vi "data_process_packet.vi"(6 "Sensor Lookup Indices":i32[](array[numeric]), 7 "Gains":dbl[](array[numeric])=[1.502, 1.502, 2.42], 8 "error in (no error)":errorcluster, 10 "No. Sensors":i32=128, 11 "Binary Input Data":string) -> (0 "error out":errorcluster, 1 "Raw Sensors N x XYZ":dbl[][](array[numeric]), 2 "Raw Sensors (Flattened)":i16[](array[numeric]), 3 "Time":u32, 4 "Sensors (uT)":dbl[][](array[numeric]))   [LabVIEW 2018]
panel:
  in  "LE?":bool=TRUE
  out "index of element":i32
  in  "threshold":dbl
  out "Z data":dbl[](graph)
  in  "byte order (0:big-endian, network order)":T1(ring)=enum."little-endian"
  out "Time Packet":string
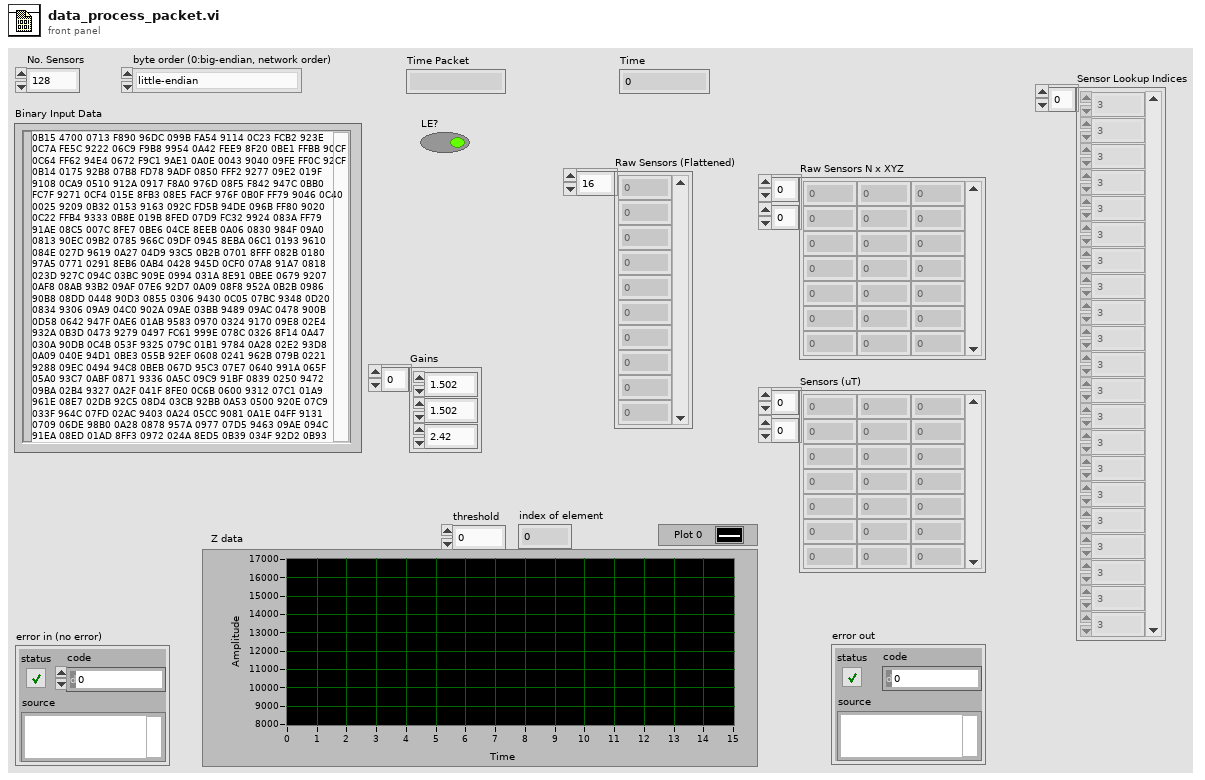
[diagram p1: front panel]
types:
  T1 = enum16{"big-endian, network order", "native, host order", "little-endian"}
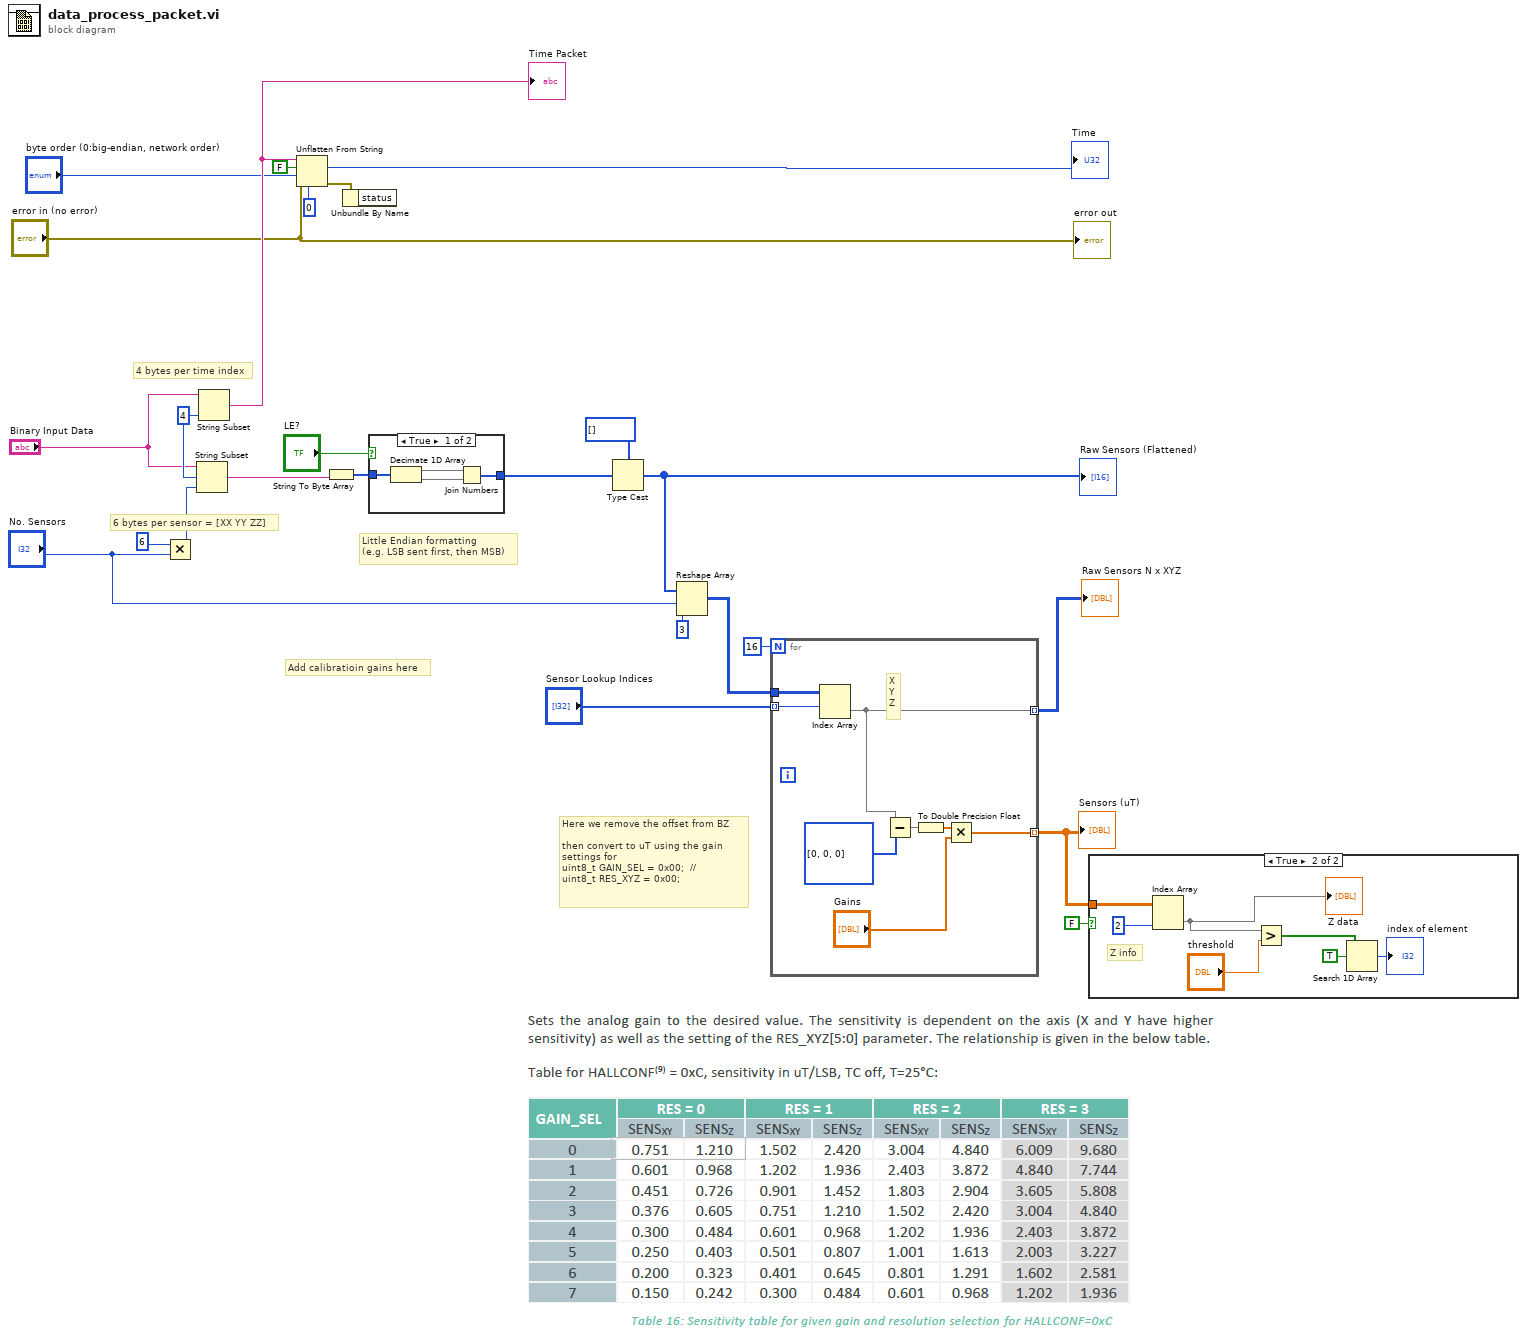
[diagram p0: block diagram]
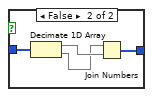
[diagram p2: hidden frame]
diagram:
  w25 = 4 ("length (rest)")
  # "Here we remove the offset from BZ\n\nthen convert to uT using the gain\nsettings for \nuint8_t GAIN_SEL = 0x00;  // \nuint8_t RES_XYZ = 0x00;"
  # "Add calibratioin gains here"
  # "4 bytes per time index"
  # "6 bytes per sensor = [XX YY ZZ]"
  # "Little Endian formatting\n(e.g. LSB sent first, then MSB)"
  n1 = Multiply(x=6 ("length (rest)"), y="No. Sensors") -> (x*y=w13:i32)
  n2 = String Subset(string="Binary Input Data", offset (0)=w25, length (rest)=w13) -> (substring=w3:string)
  n3 = String Subset(string="Binary Input Data", length (rest)=w25) -> (substring=w24:string)  [unwired: 1 in]
  "Time Packet" <- w24
  n4 = Unflatten From String(type=u32 0 ("default (0 U32)"), binary string=w24, data includes array or string size? (T)=FALSE, byte order (0:big-endian, network order)="byte order (0:big-endian, network order)", error in (no error)="error in (no error)") -> (value=→"Time":u32, error out=w17:errorcluster)  [unwired: 1 out]
  n5 = String To Byte Array(string=w3) -> (unsigned byte array=w22:u8[])
  n6 = Unbundle By Name(w17) -> ()  [unwired: 1 out]
  n7 = case shown="True" "LE?" {
    tunnel: w22 -> [w29 w33]
    tunnel: [w26 w32] -> w1
    frame True {
      n8 = Decimate 1D Array(w29) -> (w28:u8[], w27:u8[])
      n9 = Join Numbers(hi=w28, lo=w27) -> ((hi.lo)=w26:u16[])
    }
    frame False {
      n10 = Decimate 1D Array(w33) -> (w31:u8[], w30:u8[])
      n11 = Join Numbers(hi=w30, lo=w31) -> ((hi.lo)=w32:u16[])
    }
  }
  n12 = Type Cast(type=i16[] [], x=w1) -> (*(type *) &x=w12:i16[])
  "Raw Sensors (Flattened)" <- w12
  n13 = Reshape Array(w12, "No. Sensors", 3 ("milliseconds to wait")) -> (w10:i16[][])
  n14 = for {
    N: 16 -> [_]
    tunnel: w10 -> [w41]
    tunnel: [w40] -> w9 mode=indexing
    tunnel: [w35] -> w7 mode=indexing
    tunnel: "Sensor Lookup Indices" -> [w34] mode=indexing
    # "X\nY \nZ"
    n15 = Index Array(array=w41, index (row)=w34) -> (element=w40:i16[])  [unwired: 1 in]
    n16 = Subtract(x=w40, y=i16[] [0, 0, 0]) -> (x-y=w38:i16[])
    n17 = To Double Precision Float(number=w38) -> (double precision float=w37:dbl[])
    n18 = Multiply(x=w37, y="Gains") -> (x*y=w35:dbl[])
  }
  "Raw Sensors N x XYZ" <- w9
  "Sensors (uT)" <- w7
  n19 = case shown="True" FALSE {
    tunnel: w7 -> [_ w48]
    frame False {
    }
    frame True {
      # "Z info"
      n20 = Index Array(array=w48, index (col)=2 ("disabled index (col)")) -> (element=w45:dbl[])  [unwired: 1 in]
      "Z data" <- w45
      n21 = Greater?(x=w45, y="threshold") -> (0:w44:bool[])
      n22 = Search 1D Array(1D array=w44, element=TRUE) -> (index of element=→"index of element":i32)  [unwired: 1 in]
    }
  }
  "error out" <- "error in (no error)"
